vi "integal_return.vi"(0 "servo 3 dropfront":u8, 1 "servo 3 pickBack":u8) -> ()   [LabVIEW 2017]
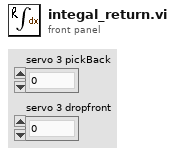
[diagram p1: front panel]
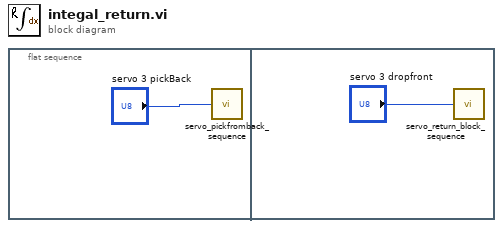
[diagram p0: block diagram]
diagram:
  n1 = flat-sequence {
    frame #0 {
      n2 = call "servo_pickfromback_sequence.vi"("pick_pos"="servo 3 pickBack") -> ()
    }
    frame #1 {
      n3 = call "servo_return_block_sequence.vi"("servo 3"="servo 3 dropfront") -> ()
    }
  }
